vi "Actor Core.vi"(8 "error in":errorcluster, 11 "Launch IMAQ Display in":refnum<class "Launch IMAQ Display.lvclass">) -> (0 "error out":errorcluster, 3 "Actor out":refnum<class "Actor.lvclass">)   [LabVIEW 2014, in "Launch IMAQ Display.lvlib" / "Launch IMAQ Display.lvclass"]
doc: "(<B>Filename</B>: Actor Framework.lvlib:Actor.lvclass:Actor Core.vi)\n\nReceives messages to the actor, reacts to them, and initiates any error handling that may shut the actor down.\n\nDescendant classes may override this VI to append parallel tasks for the actor to complete while it handles messages. Overrides use the Call Parent Method node."
uses:
  Launch IMAQ Display.lvclass
  <vilib>/ActorFramework/Actor/Actor.lvclass
  Display Actors/HIJ IMAQdx Display/AF IMAQ Display/HIJ IMAQdx Display.lvclass
  Analyze/Analyze Classes/Analyze Diviation/Analyze BeamDeviation.lvclass
  Analyze/Results and Overlays/Results Beam Deviation/Analyze Results Beam Deviation.lvclass
  Analyze/Analyze Classes/Analyze Distanz/Analyze Distanz.lvclass
  Analyze/Results and Overlays/Results Distance/Analyze Results Distanz.lvclass
  Camera Actors/IMAQdx Actor/IMAQdx Actor/IMAQdx Actor.lvclass
  Analyze/Analyze Classes/Analyze Fluence/Analyze Fluence.lvclass
  Analyze/Results and Overlays/Results Fluence/Analyze Results Fluence.lvclass
  Analyze/Analyze Parameter/Analyze Parameter Energy/Analyze Parameter Energy.lvclass
  Analyze/Analyze Parameter/Analyze Parameter Fluence/Analyze Parameter Fluence.lvclass
  Analyze/Results and Overlays/Results Base/Analyze Results Base.lvclass/Analyze Results Base.ctl
  Display Actors/HIJ Vision Display/HIJ Vision Display/HIJ Vision Display.lvclass/HIJ Vision Display.ctl
  Analyze/Analyze Parameter/Analyze Parameter Energy/Analyze Parameter Energy.lvclass/Analyze Parameter Energy.ctl
  Analyze/Results and Overlays/Results Fluence/Analyze Results Fluence.lvclass/Analyze Results Fluence.ctl
  HIJ Vision Application/HIJ Vision Application/HIJ Vision Application.lvclass/HIJ Vision Application.ctl
  HIJ Vision Camera App/HIJ Vision Camera App/HIJ Vision Camera App.lvclass/HIJ Vision Camera App.ctl
  <vilib>/ActorFramework/Actor/Actor.lvclass/Actor.ctl
  <vilib>/ActorFramework/Message Enqueuer/Message Enqueuer.lvclass/Message Enqueuer.ctl
  HIJ Vision Camera App/HIJ Vision Camera App Messages/Menu Selection Msg/Menu Selection Msg.lvclass/Menu Selection Msg.ctl
  HIJ Vision Application/HIJ Vision Application Messages/Set Parameter Msg/Set Parameter Msg.lvclass/Set Parameter Msg.ctl
  Analyze/Analyze Parameter/Analyze Parameter Energy/Write Energy.vi
  Analyze/Results and Overlays/Results Base/Write Overlay colors.vi
  Analyze/Results and Overlays/Results Base/Write Overlay_.vi
  Analyze/Results and Overlays/Results Fluence/Write UI Ref Max F.vi
  Display Actors/HIJ Vision Display/HIJ Vision Display/Write Save Report_.vi
  HIJ Vision Application/HIJ Vision Application/Write SubPnl for Display.vi
  HIJ Vision Camera App/HIJ Vision Camera App/Write Child Menu.vi
  HIJ Vision Application/HIJ Vision Application/Write HIJ Vision Display.vi
  HIJ Vision Application/HIJ Vision Application/Write Analyze Objs.vi
  HIJ Vision Camera App/HIJ Vision Camera App/Write Camera Actor.vi
  HIJ Vision Camera App/HIJ Vision Camera App/Write SubPnl for Settings.vi
  <vilib>/ActorFramework/Message Enqueuer/Init from Existing Queue.vi
  <vilib>/ActorFramework/Message Enqueuer/Enqueue.vi
  Analyze/Analyze Classes/Analyze BaseClass/Analyze BaseClass/Set Result Settings.vi
  Analyze/Analyze Classes/Analyze BaseClass/Analyze BaseClass/Set Parameter.vi
  <vilib>/ActorFramework/Message Priority Queue/Priority Enqueue.vi
  <vilib>/ActorFramework/Message Enqueuer/Message Enqueuer.lvclass
  HIJ Vision Camera App/HIJ Vision Camera App Messages/Menu Selection Msg/Menu Selection Msg.lvclass
  HIJ Vision Application/HIJ Vision Application Messages/Set Parameter Msg/Set Parameter Msg.lvclass
  <vilib>/ActorFramework/Stop Msg/Stop Msg.lvclass
  HIJ Vision Camera App/HIJ Vision Camera App/HIJ Vision Camera App.lvclass
panel:
  in  "Energy":dbl[unit]=10.0
  out "Max Fluence":dbl[unit]
  in  "Stop Button":bool
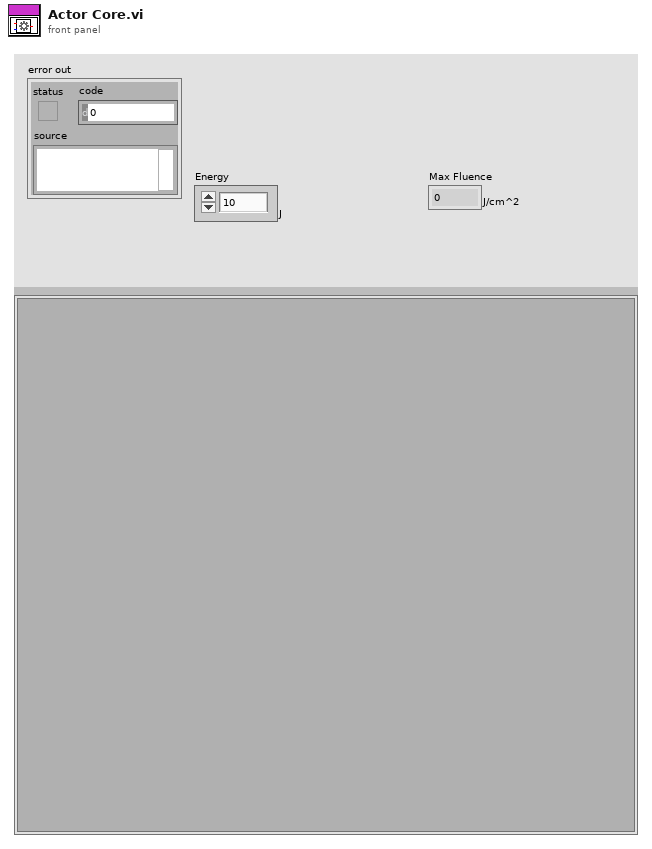
[diagram p1: front panel]
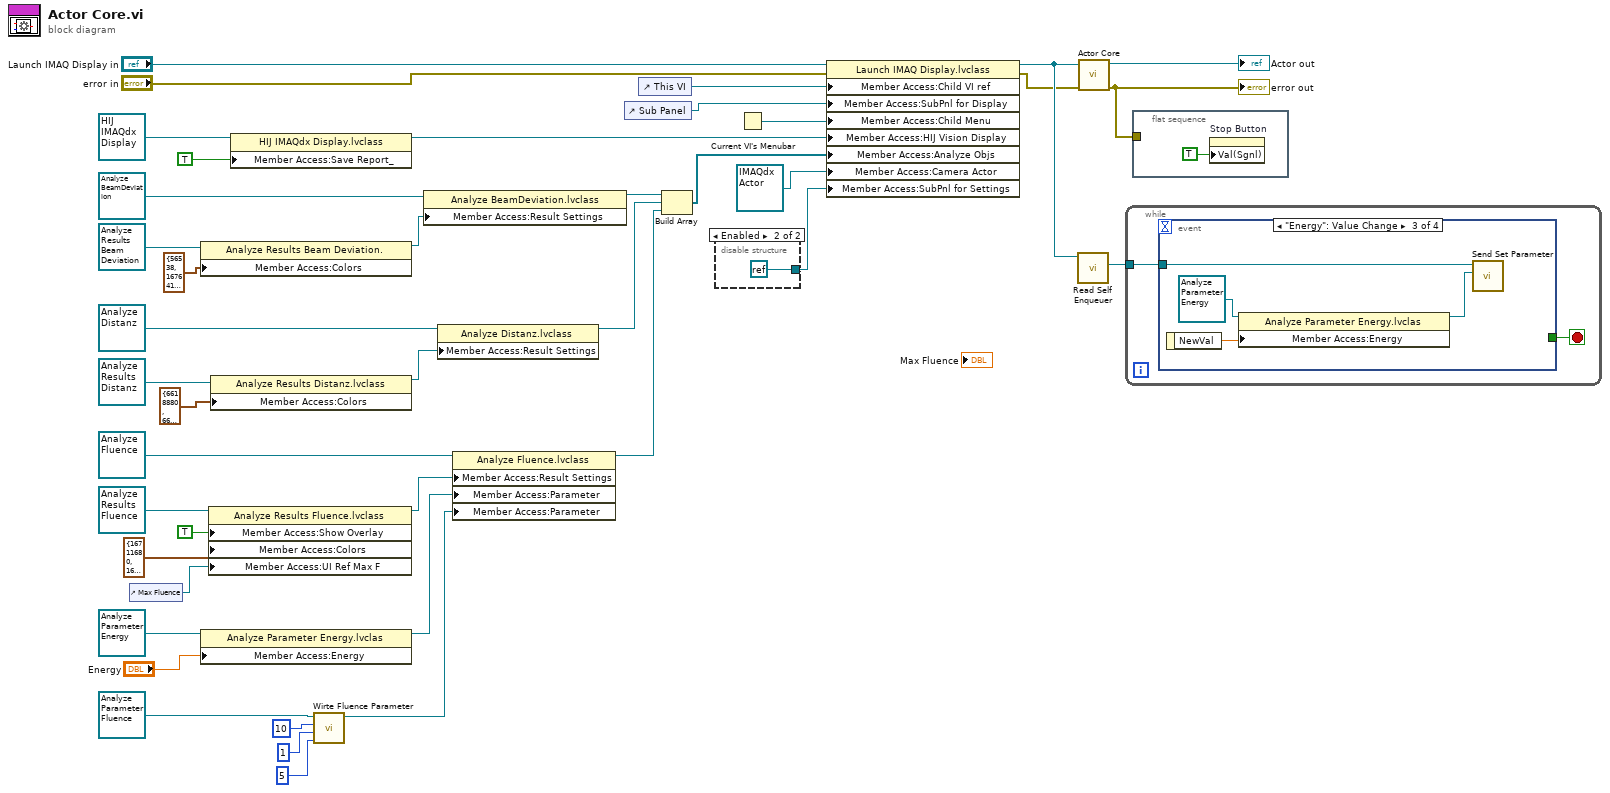
[diagram p0: block diagram]
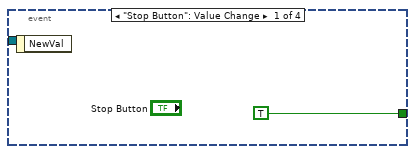
[diagram p3: hidden frame]
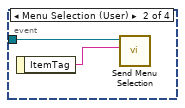
[diagram p4: hidden frame]
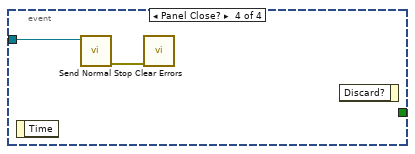
[diagram p5: hidden frame]
diagram:
  n1 = control-ref of="Max Fluence"() -> (w15:refnum<vi>)
  n2 = property class="Analyze Results Beam Deviation."(reference=refnum<class "Analyze Results Beam Deviation.lvclass"> refnum ("Analyze Results Beam Deviation.lvclass"), "Member Access:Colors"=cluster{"Border":u32, "Text":u32} {"Border"=56538, "Text"=16764160} ("Colors")) -> (reference out=w12:refnum<class "Analyze Results Beam Deviation.lvclass">)  [unwired: 1 in, 1 out]
  n3 = property class="Analyze Parameter Energy.lvclas"(reference=refnum<class "Analyze Parameter Energy.lvclass"> refnum ("Analyze Parameter Energy.lvclass"), "Member Access:Energy"="Energy") -> (reference out=w8:refnum<class "Analyze Parameter Energy.lvclass">)  [unwired: 1 in, 1 out]
  n4 = property class="Analyze Results Fluence.lvclass"(reference=refnum<class "Analyze Results Fluence.lvclass"> refnum ("Analyze Results Fluence.lvclass"), "Member Access:Show Overlay"=TRUE ("bOverlay"), "Member Access:Colors"=cluster{"Border":u32, "Text":u32} {"Border"=16711680, "Text"=16448250} ("Colors"), "Member Access:UI Ref Max F"=w15) -> (reference out=w14:refnum<class "Analyze Results Fluence.lvclass">)  [unwired: 1 in, 1 out]
  n5 = property class="Analyze Results Distanz.lvclass"(reference=refnum<class "Analyze Results Distanz.lvclass"> refnum ("Analyze Results Distanz.lvclass"), "Member Access:Colors"=cluster{"Border":u32, "Text":u32} {"Border"=6618880, "Text"=6618880} ("Colors")) -> (reference out=w11:refnum<class "Analyze Results Distanz.lvclass">)  [unwired: 1 in, 1 out]
  n6 = property class="HIJ IMAQdx Display.lvclass"(reference=refnum<class "HIJ IMAQdx Display.lvclass"> refnum ("IMAQ Display.lvlib:IMAQ Display.lvclass"), "Member Access:Save Report_"=TRUE ("Save Report_")) -> (reference out=w21:refnum<class "HIJ IMAQdx Display.lvclass">)  [unwired: 1 in, 1 out]
  n7 = call "Wirte Fluence Parameter.vi"("#of Areas"=5, "#Overlays"=1, "Size of region (px)"=10, "Analyze Parameter Fluence in"=refnum<class "Analyze Parameter Fluence.lvclass"> refnum ("Analyze Parameter Fluence.lvclass")) -> ("Analyze Parameter Fluence out"=w6:refnum<class "Analyze Parameter Fluence.lvclass">)  [unwired: 7 in]
  n8 = property class="Analyze BeamDeviation.lvclass"(reference=refnum<class "Analyze BeamDeviation.lvclass"> refnum ("Analyze.lvlib:Analyze BeamDeviation.lvclass"), "Member Access:Result Settings"=w12) -> (reference out=w13:refnum<class "Analyze BeamDeviation.lvclass">)  [unwired: 1 in, 1 out]
  n9 = property class="Analyze Distanz.lvclass"(reference=refnum<class "Analyze Distanz.lvclass"> refnum ("Analyze.lvlib:Analyze Distanz.lvclass"), "Member Access:Result Settings"=w11) -> (reference out=w2:refnum<class "Analyze Distanz.lvclass">)  [unwired: 1 in, 1 out]
  n10 = property class="Analyze Fluence.lvclass"(reference=refnum<class "Analyze Fluence.lvclass"> refnum ("Analyze.lvlib:Analyze Fluence.lvclass"), "Member Access:Result Settings"=w14, "Member Access:Parameter"=w8, "Member Access:Parameter"=w6) -> (reference out=w1:refnum<class "Analyze Fluence.lvclass">)  [unwired: 1 in, 1 out]
  n11 = control-ref of="Sub Panel"() -> (w24:refnum<vi>)
  n12 = control-ref of="This VI"() -> (w28:refnum<vi>)
  n13 = Build Array(w13, w2, w1) -> (w25:refnum<class "Analyze BaseClass.lvclass">[])
  n14 = disable-structure shown="Enabled" {
    disable-tunnel: [_ refnum<k0> refnum] -> w22
    frame Disabled {
    }
    frame Enabled {
    }
  }
  n15 = Current VI's Menubar() -> (w20:refnum<k9>)
  n16 = property class="Launch IMAQ Display.lvclass"(reference="Launch IMAQ Display in", error in="error in", "Member Access:Child VI ref"=w28, "Member Access:SubPnl for Display"=w24, "Member Access:Child Menu"=w20, "Member Access:HIJ Vision Display"=w21, "Member Access:Analyze Objs"=w25, "Member Access:Camera Actor"=refnum<class "IMAQdx Actor.lvclass"> refnum ("IMAQdx Actor.lvlib:IMAQdx Actor.lvclass"), "Member Access:SubPnl for Settings"=w22) -> (reference out=w29:refnum<class "Launch IMAQ Display.lvclass">, error out=w26:errorcluster)
  n17 = call <vilib>:"Read Self Enqueuer.vi"("Actor"=w29) -> ("Self Enqueuer"=w38:refnum<class "Message Enqueuer.lvclass">)  [unwired: 10 in]
  n18 = call-parent "Actor Core.vi"("error in"=w26, "Launch IMAQ Display in"=w29) -> ("error out"=w39:errorcluster, "Actor out"=→"Actor out":refnum<class "Actor.lvclass">)  [unwired: 8 in]
  "error out" <- w39
  n19 = while {
    tunnel: w38 -> [w43]
    stop <- w44 stop-if-true
    n20 = event shown="[2] \"Energy\": Value Change" {
      selector: _ -> [_ _ _ _]
      dyn-events: _ -> [_ _ _ _]
      timeout: _ -> [_ _ _ _]
      tunnel: [TRUE _ _ _] -> w44
      tunnel: w43 -> [_ w46 w49 w53]
      event "Stop Button": Value Change {
        n21 = event-data() -> ()  [unwired: 1 in, 1 out]
      }
      event Menu Selection (User) {
        n22 = event-data() -> ("ItemTag"=w47:string)  [unwired: 1 in]
        n23 = call "Send Menu Selection.vi"("MenuTag"=w47, "Message Enqueuer"=w46) -> ()  [unwired: 8 in, 2 out]
      }
      event "Energy": Value Change {
        n24 = event-data() -> ("NewVal"=w50:dbl[unit])  [unwired: 1 in]
        n25 = property class="Analyze Parameter Energy.lvclas"(reference=refnum<class "Analyze Parameter Energy.lvclass"> refnum ("Analyze Parameter Energy.lvclass"), "Member Access:Energy"=w50) -> (reference out=w48:refnum<class "Analyze Parameter Energy.lvclass">)  [unwired: 1 in, 1 out]
        n26 = call "Send Set Parameter.vi"("Parameter"=w48, "Message Enqueuer"=w49) -> ()  [unwired: 8 in, 2 out]
      }
      event Panel Close? {
        n27 = event-data() -> ()  [unwired: 1 in, 1 out]
        n28 = call <vilib>:"Send Normal Stop.vi"("Message Enqueuer"=w53) -> ("error out"=w52:errorcluster)  [unwired: 10 in]
        n29 = call <vilib>:"Clear Errors.vi"("error in (no error)"=w52) -> ()  [unwired: 5 in, 2 out]
        n30 = event-data() -> ()  [unwired: 2 in, 1 out]
      }
    }
  }
  n31 = flat-sequence {
    tunnel: w39 -> [_]
    frame #0 {
      n32 = property on="Stop Button" class="Bool (strict)"("Val(Sgnl)"=TRUE) -> ()  [unwired: 2 in, 2 out]
    }
  }
